vi "Start Beacon.vi"(0 "name":string, 5 "TCP Server EndPoint":T1) -> (15 "error out":errorcluster)   [LabVIEW 2020, in "epl-network.lvlib"]
uses:
  epl-network.lvlib
  TCP/Typedefs/IPEndPoint.ctl
  Private/Beacon FGV.ctl
  Private/Discovery Beacon Broadcast Loop.vi
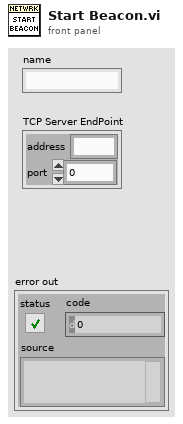
[diagram p1: front panel]
types:
  T1 = typedef "epl-network.lvlib/IPEndPoint.ctl" = cluster{"address":string, "port":i32}
  T2 = typedef "epl-network.lvlib/Beacon FGV.ctl" = cluster{"receiver":refnum<vi>, "stop":refnum<notifier>}
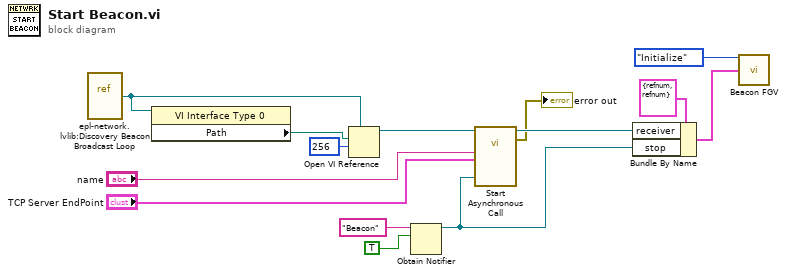
[diagram p0: block diagram]
diagram:
  n1 = vi-ref "epl-network.lvlib:Discovery Beacon Broadcast Loop.vi"() -> (w8:refnum<vi>)
  n2 = property class="VI Interface Type 0"(reference=w8) -> ("Path"=w9:path)  [unwired: 1 in, 2 out]
  n3 = Open VI Reference(type specifier VI Refnum (for type only)=w8, vi path=w9, options=256) -> (vi reference=w10:refnum<vi>)  [unwired: 3 in, 1 out]
  n4 = Obtain Notifier(name (unnamed)="Beacon", notification data type=TRUE) -> (notifier out=w2:refnum<notifier>)  [unwired: 2 in, 2 out]
  n5 = call-by-ref "Start Asynchronous Call"(reference=w10, "name"="name", "TCP Server EndPoint"="TCP Server EndPoint", "kill thread notifier"=w2) -> (reference out=w5:refnum<vi>, error out=→"error out":errorcluster)  [unwired: 14 in]
  n6 = Bundle By Name(cluster=T2 {"receiver"=refnum, "stop"=refnum} ("data in"), "receiver"=w5, "stop"=w2) -> (w6:T2)
  n7 = call "Beacon FGV.vi"("action"=enum16{"Initialize", "Get"}."Initialize", "data in"=w6) -> ()  [unwired: 13 in, 1 out]
